vi "make graphs_focus stack method.vi"(8 "error in (no error)":errorcluster, 11 "Autofocus in":refnum<class "Autofocus.lvclass">) -> (0 "error out":errorcluster, 1 "Latest Focus curve":T1(graph), 2 "Linear fit through stack":T2(graph), 3 "Autofocus out":refnum<class "Autofocus.lvclass">)   [LabVIEW 2012, in "Autofocus.lvclass"]
uses:
  Autofocus.lvclass
  Autofocus.lvclass/Autofocus.ctl
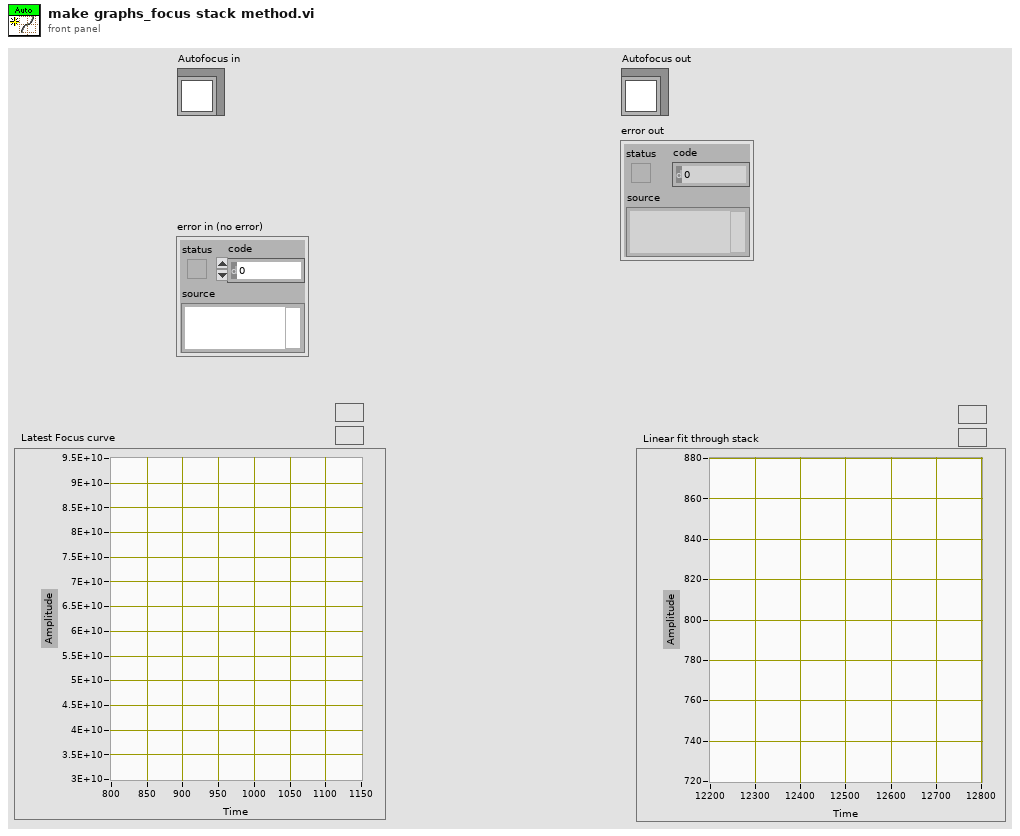
[diagram p1: front panel]
types:
  T1 = cluster{"defocus positions to graph":dbl[], "gaussian fit to graph":dbl[]}[]
  T2 = cluster{"stage positions":dbl[], "focus positions":dbl[]}[]
  T3 = cluster{"stage positions":dbl[], "focus positions":dbl[]}
  T4 = cluster{"stage positions":dbl[], "best linear fit":dbl[]}
  T5 = cluster{"defocus positions to graph":dbl[], "Image sharpness array to graph":dbl[]}
  T6 = cluster{"defocus positions to graph":dbl[], "gaussian fit to graph":dbl[]}
  T7 = cluster{"stage positions":dbl[], "best linear fit":dbl[]}[]
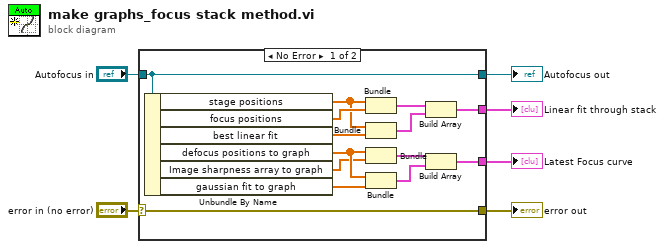
[diagram p0: block diagram]
diagram:
  n1 = case shown="No Error" "error in (no error)" {
    selector: "error in (no error)" -> [w20 w22]
    tunnel: [w20 w22] -> w5
    tunnel: [w14 w21] -> w3
    tunnel: "Autofocus in" -> [w14 w21]
    tunnel: [w17 _] -> w2
    tunnel: [w16 _] -> w1
    frame No Error {
      n2 = Unbundle By Name(w14) -> ("stage positions"=w12:dbl[], "focus positions"=w13:dbl[], "best linear fit"=w11:dbl[], "defocus positions to graph"=w10:dbl[], "Image sharpness array to graph"=w9:dbl[], "gaussian fit to graph"=w8:dbl[])
      n3 = Bundle("stage positions"=w12, "focus positions"=w13) -> (w19:T3)  [unwired: 1 in]
      n4 = Bundle("stage positions"=w12, "best linear fit"=w11) -> (w18:T4)  [unwired: 1 in]
      n5 = Bundle("defocus positions to graph"=w10, "Image sharpness array to graph"=w9) -> (w15:T5)  [unwired: 1 in]
      n6 = Bundle("defocus positions to graph"=w10, "gaussian fit to graph"=w8) -> (w7:T6)  [unwired: 1 in]
      n7 = Build Array(w19, w18) -> (w17:T7)
      n8 = Build Array(w15, w7) -> (w16:T1)
    }
    frame Error {
    }
  }
  "error out" <- w5
  "Autofocus out" <- w3
  "Latest Focus curve" <- w1
  "Linear fit through stack" <- w2
